vi "test1.vi"() -> ()   [LabVIEW 2010]
panel:
  out "error out":errorcluster
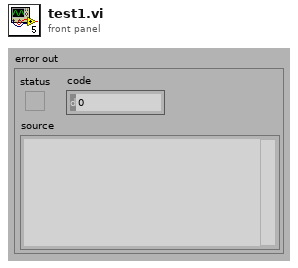
[diagram p1: front panel]
types:
  T1 = cluster{"DeviceID":i32, "DateTime":timestamp, "Files":cluster{"FileType":string, "FilePath":path}[], "Strings":string[][]}
  T2 = typedef "LVDateTimeRec.ctl" = cluster{"fractional second":dbl, "second":i32, "minute":i32, "hour":i32, "day of month":i32, "month":i32, "year":i32, "day of week":i32, "day of year":i32, "DST":i32}
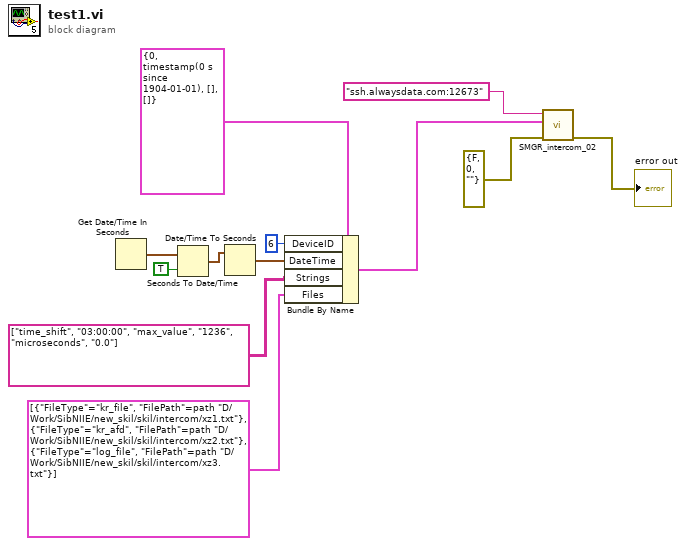
[diagram p0: block diagram]
diagram:
  n1 = Get Date/Time In Seconds() -> (seconds since 1Jan1904=w7:timestamp)
  n2 = Seconds To Date/Time(time stamp (now)=w7, to UTC (F)=TRUE) -> (date time rec=w8:T2)
  n3 = Date/Time To Seconds(2:w8) -> (0:w6:timestamp)  [unwired: 1 in]
  n4 = Bundle By Name(cluster=T1 {"DeviceID"=0, "DateTime"=timestamp(0 s since 1904-01-01), "Files"=[], "Strings"=[]} ("InputData"), "DeviceID"=6, "DateTime"=w6, "Strings"=string[][] [["time_shift", "03:00:00"], ["max_value", "1236"], ["microseconds", "0.0"]], "Files"=cluster{"FileType":string, "FilePath":path}[] [{"FileType"="kr_file", "FilePath"=path "D:/Work/SibNIIE/new_skil/skil/intercom/xz1.txt"}, {"FileType"="kr_afd", "FilePath"=path "D:/Work/SibNIIE/new_skil/skil/intercom/xz2.txt"}, {"FileType"="log_file", "FilePath"=path "D:/Work/SibNIIE/new_skil/skil/intercom/xz3.txt"}]) -> (w3:T1)
  n5 = call "SMGR_intercom_02.vi"("error in (no error)"=errorcluster {"status"=FALSE, "code"=0, "source"=""}, "InputData"=w3, "URL:port"="ssh.alwaysdata.com:12673") -> ("error out"=→"error out":errorcluster)  [unwired: 8 in]
